vi "PID Setpoint Profile.vi"(7 "reinitialize? (F)":bool, 10 "start":bool, 11 "setpoint profile":cluster{"time (s)":dbl, "setpoint":dbl}[](array[cluster]) {"setpoint" format="%.2f"; "time (s)" format="%.3f"}) -> (1 "elapsed time (s)":dbl format="%.3f", 2 "profile complete?":bool, 3 "setpoint":dbl format="%.2f")   [LabVIEW 2019, in "control.lvlib"]
uses:
  control.lvlib
  Inputs/Inputs.lvlib
  Timer Delay/Timers.lvlib
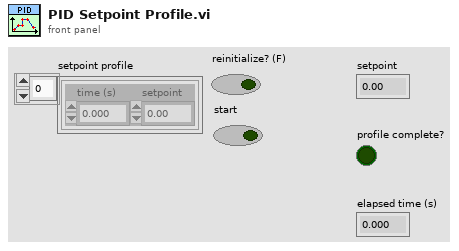
[diagram p1: front panel]
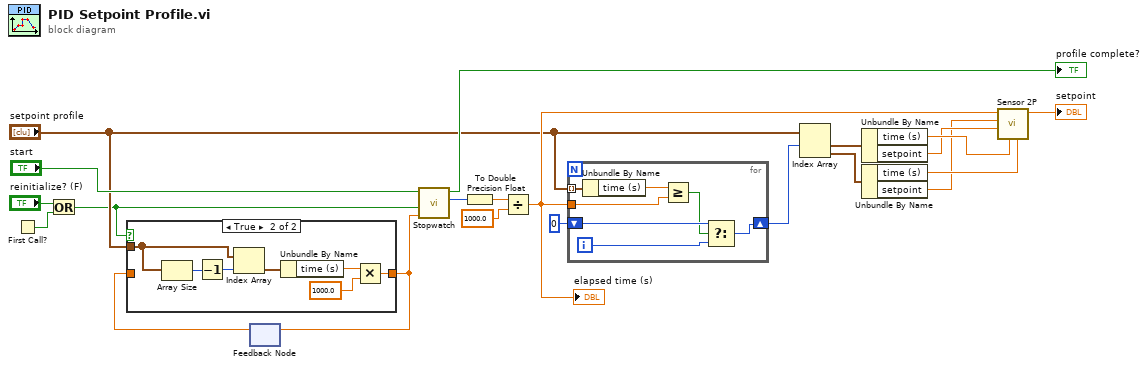
[diagram p0: block diagram]
diagram:
  n1 = First Call?() -> (First Call?: T/F=w21:bool)
  n2 = Or(x="reinitialize? (F)", y=w21) -> (x .or. y?=w9:bool)
  n3 = feedback #1() -> (w2:dbl)  [unwired: 1 in]
  n4 = case shown="True" w9 {
    tunnel: [w22 w24] -> w1
    tunnel: "setpoint profile" -> [_ w23]
    tunnel: w2 -> [w22 _]
    frame False {
    }
    frame True {
      n5 = Array Size(array=w23) -> (size(s)=w29:i32)
      n6 = Decrement(x=w29) -> (x-1=w28:i32)
      n7 = Index Array(array=w23, index=w28) -> (element=w27:cluster{"time (s)":dbl, "setpoint":dbl})
      n8 = Unbundle By Name(w27) -> ("time (s)"=w26:dbl)
      n9 = Multiply(x=w26, y=1000.0) -> (x*y=w24:dbl)
    }
  }
  n10 = feedback-in #1(w1) -> ()
  n11 = call "Stopwatch.vi"("ms"=w1, "Load"=w9, "Start"="start") -> ("t ms"=w16:u32, "End"=→"profile complete?":bool)  [unwired: 6 in]
  n12 = To Double Precision Float(number=w16) -> (double precision float=w15:dbl)
  n13 = Divide(x=w15, y=1000.0) -> (x/y=w13:dbl)
  "elapsed time (s)" <- w13
  n14 = for {
    tunnel: "setpoint profile" -> [w36] mode=indexing
    tunnel: w13 -> [w31]
    shift-right: [w35] -> w17
    shift-left: 0 -> [w34]
    i -> [w33]
    n15 = Unbundle By Name(w36) -> ("time (s)"=w32:dbl)
    n16 = Greater Or Equal?(x=w32, y=w31) -> (x >= y?=w30:bool)
    n17 = Select(t=w34, s=w30, f=w33) -> (s? t:f=w35:i32)
  }
  n18 = Index Array(array="setpoint profile", index #1=w17) -> (element #1=w8:cluster{"time (s)":dbl, "setpoint":dbl}, element #2=w7:cluster{"time (s)":dbl, "setpoint":dbl})  [unwired: 1 in]
  n19 = Unbundle By Name(w8) -> ("time (s)"=w6:dbl, "setpoint"=w5:dbl)
  n20 = Unbundle By Name(w7) -> ("time (s)"=w4:dbl, "setpoint"=w3:dbl)
  n21 = call "Sensor 2P.vi"("Xmax"=w4, "Xmin"=w6, "Ymin"=w5, "Ymax"=w3, "X"=w13) -> ("Y"=→"setpoint":dbl)  [unwired: 6 in]
